vi "总氮总磷质控流程.vi"(0 "队列输入TP":refnum<queue>, 5 "总氮量程切换":enum32{"H", "L", "AUTO"}(ring)=enum."AUTO", 7 "总磷量程切换":enum32{"H", "L", "AUTO"}(ring)=enum."AUTO", 9 "总磷":bool, 11 "总氮":bool) -> (4 "布尔":bool, 6 "总磷中断报警":bool, 8 "总氮中断报警":bool)   [LabVIEW 2016, in "质控单元.lvlib"]
panel:
  out "总磷":bool
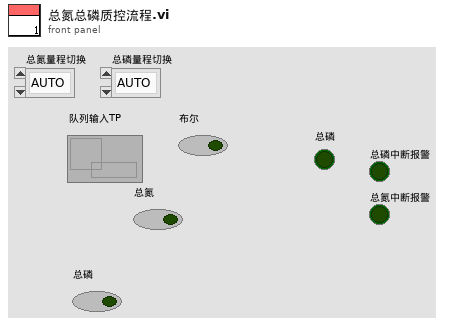
[diagram p1: front panel]
types:
  T1 = enum16{"待机", "启动氨氮水样", "氨氮测量中", "启动氨氮加标", "启动氨氮加标回收", "氨氮加标回收测量中", "启动总氮水样", "总氮测量中", "启动总氮加标", "启动总氮加标回收", "总氮加标回收测量中", "启动总磷水样", "总磷水样测量中", "启动总磷加标", "启动总磷加标回收", "总磷加标回收测量中", "结束"}
  T2 = cluster{"站号":u16, "量程切换":enum32{"H", "L", "AUTO"}, "控制命令":enum16{"启动测量", "标样核查", "零点核查", "跨度核查", "空白测试", "平行样测试", "加标回收", "空白校准", "标样校准", "初始化（清洗）", "停止测试", "仪器重启", "校时", "模式设置", "测量间隔设置"}, "模式设置":enum16{"待机", "连续模式", "周期模式", "定点模式", "受控模式", "手动模式"}, "测量间隔":u16}
  T3 = cluster{"时间标识":timestamp, "设备":string, "日志信息":string}
  T4 = cluster{"系统时间":timestamp, "工作状态":enum16{"空闲", "水样测试", "标样核查", "零点核查", "跨度核查", "空白测试", "平行样测试", "加标回收", "空白校准", "标样校准", "初始化（清洗）"}, "测量模式":enum16{"待机", "连续模式", "周期模式", "定点模式", "受控模式", "手动模式"}, "告警代码":enum16{"无告警", "缺试剂告警", "缺水样告警", "缺蒸馏水告警", "缺标液告警", "仪表漏液告警", "标定异常告警", "超量程告警", "加热异常", "低试剂预警", "超上限告警", "超下限告警", "仪表内部其他异常", "滴定异常告警", "电极异常告警", "量程切换告警", "参数设置告警", "PH电极电位异常", "电导率电极异常", "浊度光度异常", "溶解氧电极异常", "溶解氧光强异常", "温度异常告警", "PH异常告警", "溶解氧异常告警", "电导率异常告警", "浊度异常告警", "叶绿素异常告警", "藻密度异常告警", "蓝绿藻异常告警", "ORP异常告警", "氨氮异常告警", "清洁刷异常告警", "SD卡异常告警", "蓝牙异常告警", "Wifi异常告警", "流程异常告警"}, "故障代码":enum16{"无故障", "电机故障", "温度故障", "通讯故障", "滴定故障"}, "日志代码":u16, "软件版本":u16, "F0":sgl, "F1":sgl, "F2":sgl, "F3":sgl, "T":sgl, "H":sgl, "id":u16, "flowid":u16, "量程":u16, "总磷控温温度1":sgl, "营养盐控温温度2":sgl, "ADC":sgl}
  T5 = enum16{"空闲", "水样测试", "标样核查", "零点核查", "跨度核查", "空白测试", "平行样测试", "加标回收", "空白校准", "标样校准", "初始化（清洗）"}
  T6 = cluster{"因子编码":u32, "单位":u16, "标样参考值":sgl, "水样数据时间":timestamp, "水样实测值":sgl, "水样数据标识":string, "标样数据时间":timestamp, "标样实测值":sgl, "标样数据标识":string, "空白数据时间":timestamp, "空白实测值":sgl, "空白数据标识":string, "零点核查数据时间":timestamp, "零点核查实测值":sgl, "零点核查数据标识":string, "跨度核查数据时间":timestamp, "跨度核查实测值":sgl, "跨度核查数据标识":string, "加标回收数据时间":timestamp, "加标回收实测值":sgl, "加标回收数据标识":string, "平行样数据时间":timestamp, "平行样实测值":sgl, "平行样数据标识":string}
  T7 = cluster{"量程":dbl, "检出限":dbl, "加标前水样浓度":dbl, "加标后水样浓度":dbl, "加标水杯定容体积":dbl, "加标母液浓度":dbl, "加标体积":dbl, "加标回收率":dbl}
  T8 = cluster{"氨氮":u8, "总磷":u8, "总氮":u8, "CODMn":u8, "CODCr":u8}
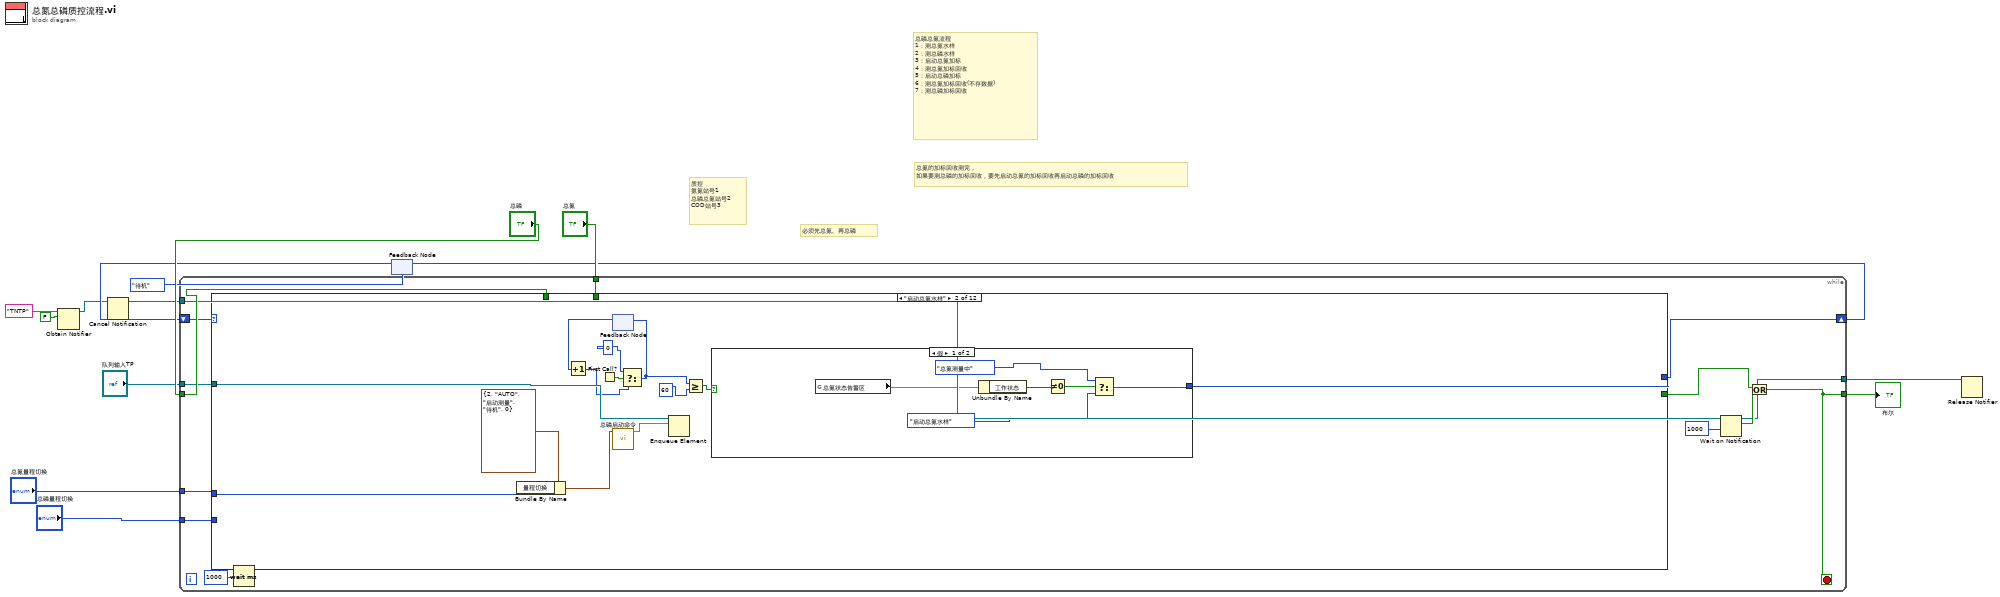
[diagram p0: block diagram]
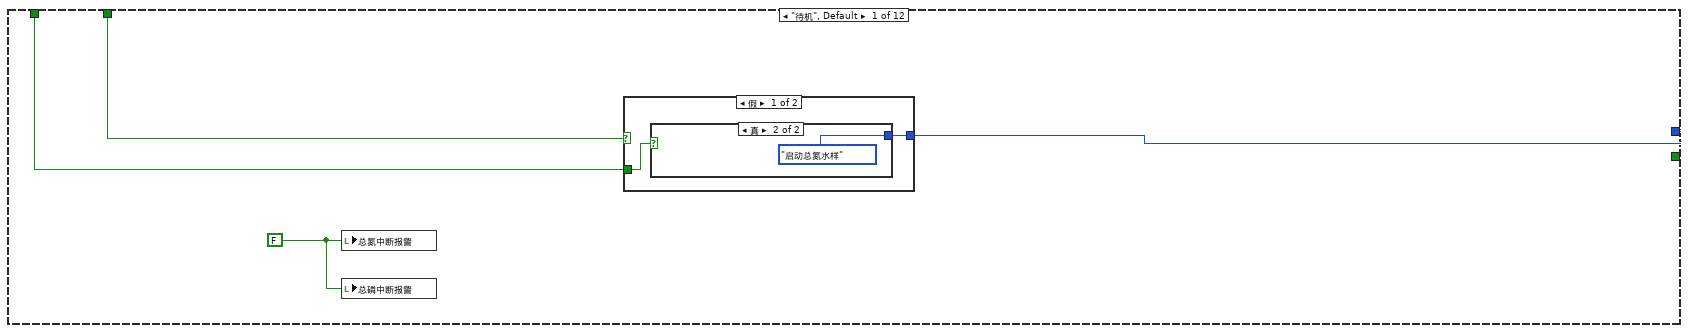
[diagram p2: hidden frame]
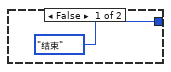
[diagram p3: hidden frame]
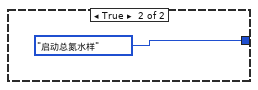
[diagram p4: hidden frame]
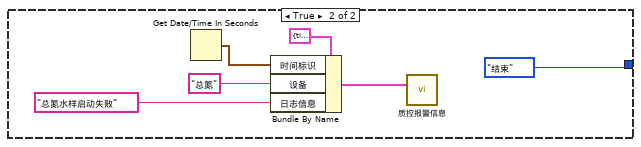
[diagram p5: hidden frame]
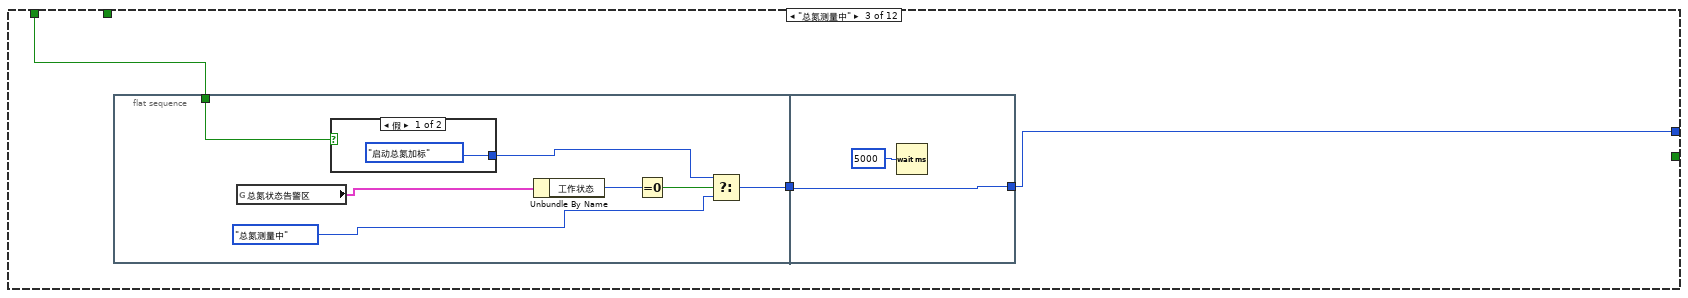
[diagram p6: hidden frame]
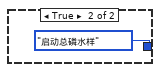
[diagram p7: hidden frame]
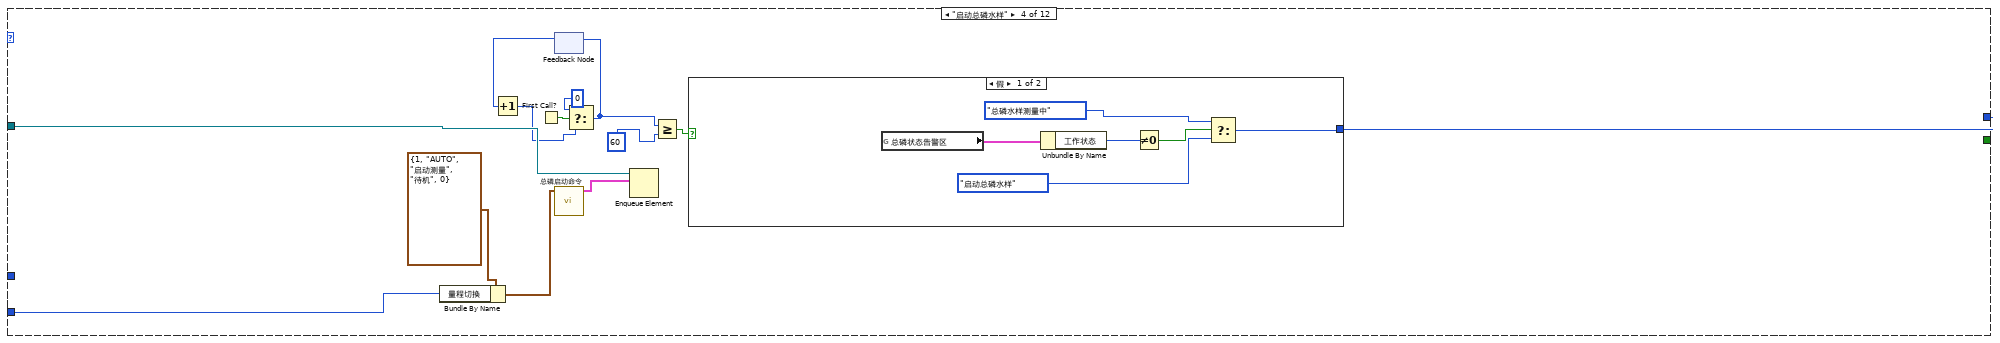
[diagram p8: hidden frame]
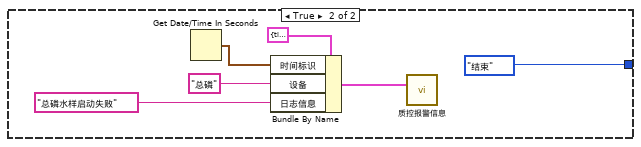
[diagram p9: hidden frame]
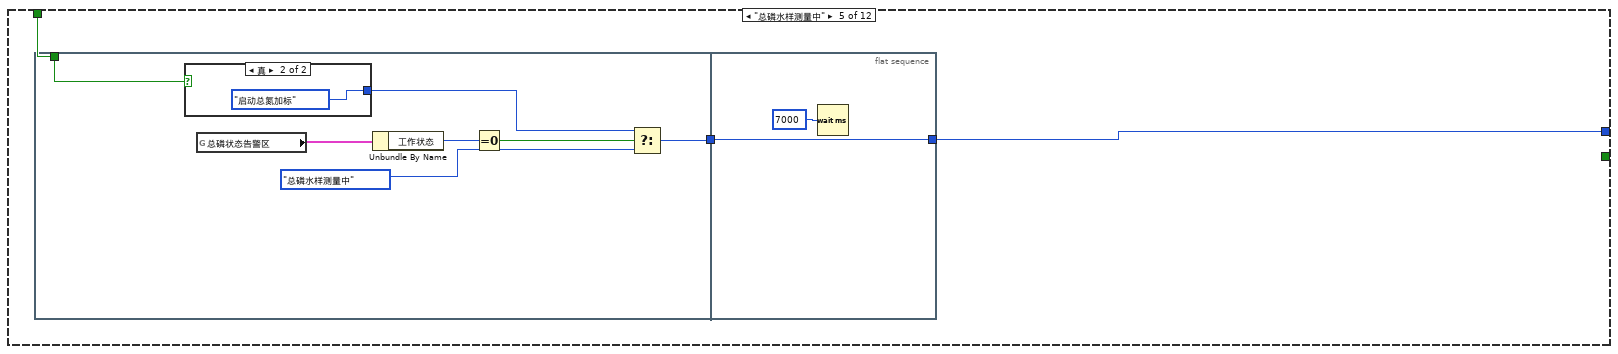
[diagram p10: hidden frame]
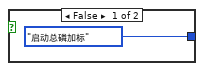
[diagram p11: hidden frame]
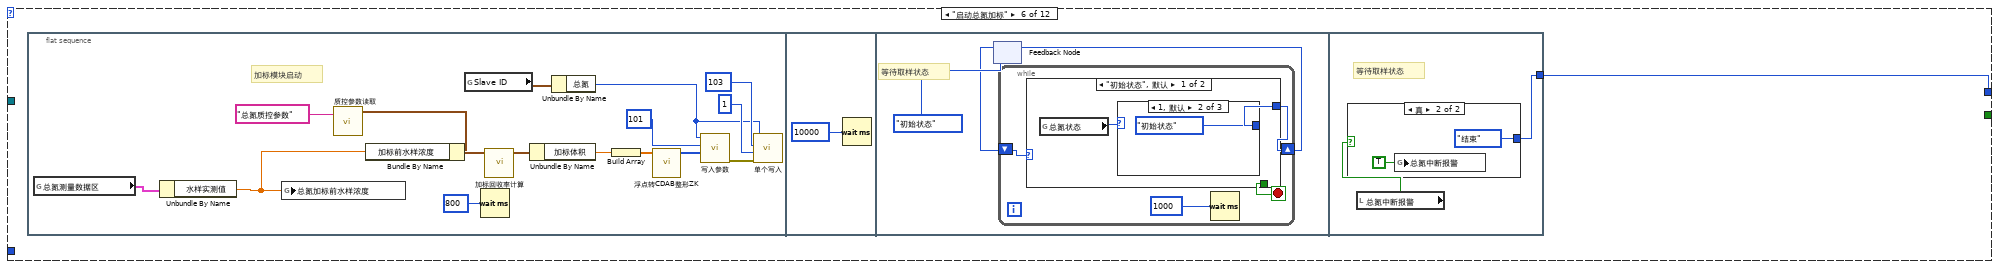
[diagram p12: hidden frame]
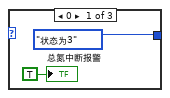
[diagram p13: hidden frame]
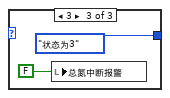
[diagram p14: hidden frame]
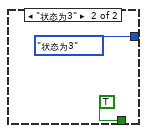
[diagram p15: hidden frame]
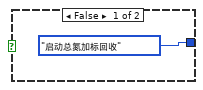
[diagram p16: hidden frame]
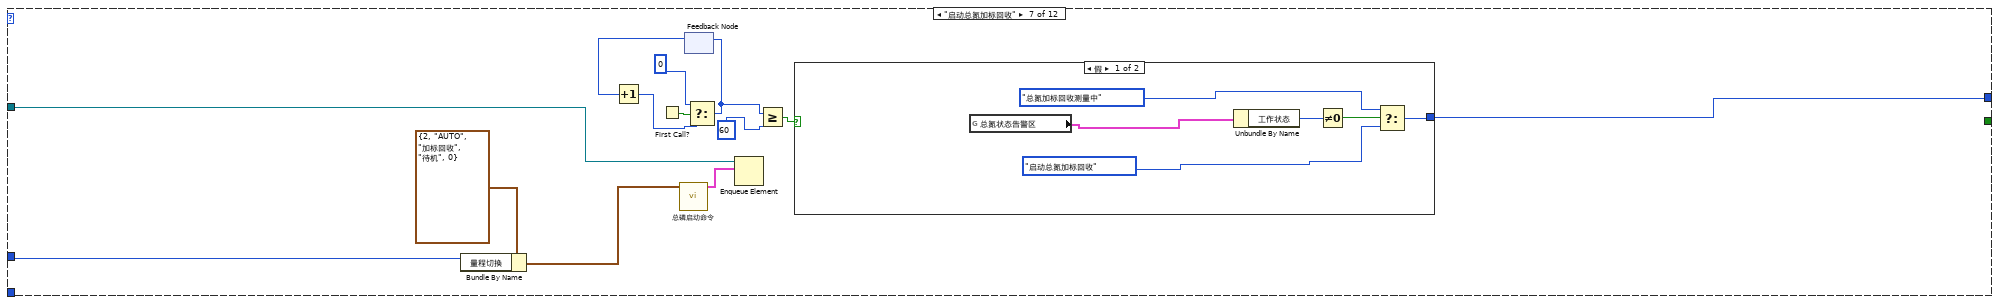
[diagram p17: hidden frame]
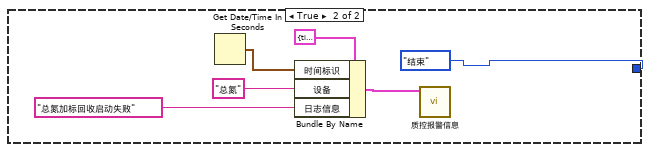
[diagram p18: hidden frame]
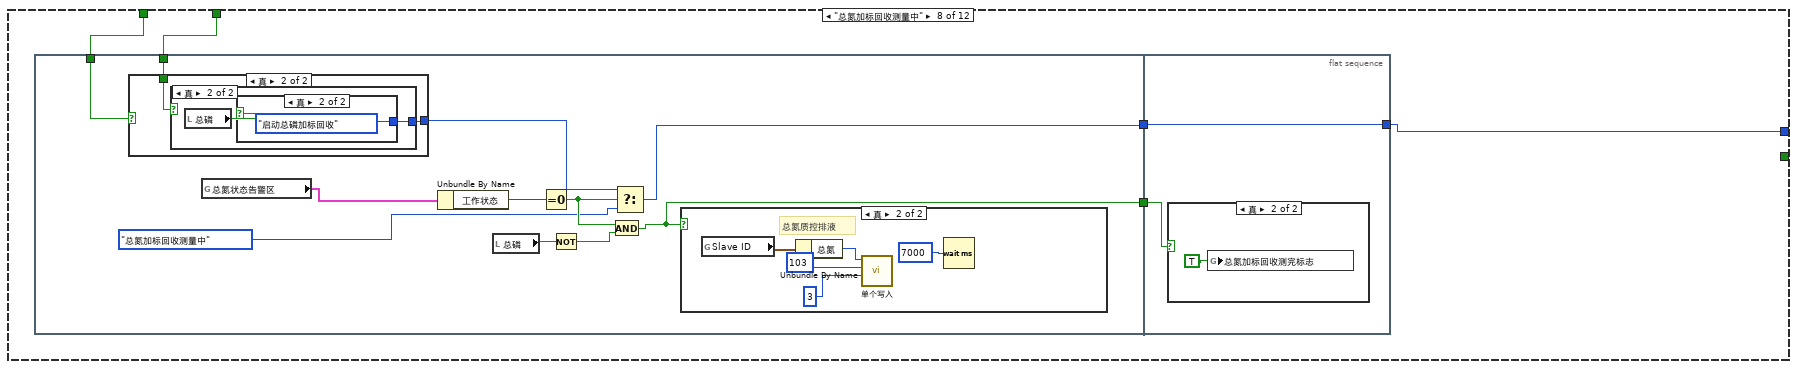
[diagram p19: hidden frame]
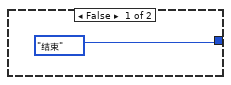
[diagram p20: hidden frame]
diagram:
  # "总磷总氮流程\n1：测总氮水样\n2：测总磷水样\n3：启动总氮加标\n4：测总氮加标回收\n5：启动总磷加标\n6：测总氮加标回收(不存数据)\n7：测总磷加标回收"
  # "总氮的加标回收测完，\n如果要测总磷的加标回收，要先启动总氮的加标回收再启动总磷的加标回收"
  # "质控\n氨氮站号1   \n总磷总氮站号2\nCOD站号3"
  # "必须先总氮、再总磷"
  n1 = Obtain Notifier(name (unnamed)="TNTP" ("名称（未命名）"), notification data type=FALSE) -> (notifier out=w3:refnum<notifier>)  [unwired: 2 in, 2 out]
  n2 = Cancel Notification(0:w3) -> (8:w2:refnum<notifier>)  [unwired: 1 in, 2 out]
  n3 = feedback #1(T1."待机") -> (w6:T1)
  n4 = while {
    tunnel: "队列输入TP" -> [w27]
    tunnel: "总氮" -> [w26]
    tunnel: "总氮量程切换" -> [w24]
    tunnel: "总磷量程切换" -> [w23]
    shift-right: [w25] -> w9
    shift-left: w6 -> [w22]
    tunnel: "总磷" -> [w28]
    tunnel: [w18] -> w13
    tunnel: w2 -> [w17]
    tunnel: [w16] -> w1
    stop <- w18 stop-if-true
    n5 = case shown="\"启动总氮水样\"" w22 {
      tunnel: [w32 w49 w64 w88 w104 w116 w158 w182 w212 w257 w280 T1."结束"] -> w25
      tunnel: w27 -> [_ w50 _ w89 _ _ w160 _ _ w258 _ _]
      tunnel: [_ _ _ _ _ _ _ _ _ _ _ TRUE] -> w19
      tunnel: w28 -> [w31 _ w63 _ _ _ _ w183 _ _ _ _]
      tunnel: w26 -> [w30 _ _ _ w102 _ _ w181 _ _ _ _]
      tunnel: w24 -> [_ w38 _ _ _ _ w155 _ _ _ _ _]
      tunnel: w23 -> [_ _ _ w77 _ _ _ _ _ w253 _ _]
      frame "待机", Default {
        w29 = FALSE ("总氮中断报警")
        n6 = local write "总氮中断报警"(w29) -> ()
        n7 = local write "总磷中断报警"(w29) -> ()
        n8 = case shown="假" w30 {
          tunnel: w31 -> [w33 _]
          tunnel: [w34 T1."启动总氮水样"] -> w32
          frame False {
            n9 = case shown="真" w33 {
              tunnel: [T1."结束" T1."启动总氮水样"] -> w34
              frame False {
              }
              frame True {
              }
            }
          }
          frame True {
          }
        }
      }
      frame "启动总氮水样" {
        n10 = Bundle By Name(cluster=T2 {"站号"=2, "量程切换"=enum."AUTO", "控制命令"=enum."启动测量", "模式设置"=enum."待机", "测量间隔"=0} ("参数"), "量程切换"=w38) -> (w39:T2)
        n11 = First Call?() -> (First Call?: T/F=w47:bool)
        n12 = feedback #2() -> (w46:i32)  [unwired: 1 in]
        n13 = Increment(x=w46) -> (x+1=w45:i32)
        n14 = call "总磷启动命令.vi"("参数"=w39) -> ("启动命令"=w41:cluster{"命令":string, "data":variant})  [unwired: 10 in]
        n15 = Select(t=0, s=w47, f=w45) -> (s? t:f=w44:i32)
        n16 = feedback-in #2(w44) -> ()
        n17 = Enqueue Element(queue=w50, element=w41) -> ()  [unwired: 2 in, 3 out]
        n18 = Greater Or Equal?(x=w44, y=60) -> (x >= y?=w42:bool)
        n19 = case shown="假" w42 {
          tunnel: [w54 T1."结束"] -> w49
          frame False {
            n20 = global read "与总氮交互全局.vi" "总氮状态告警区"() -> (w51:T4)
            n21 = Unbundle By Name(w51) -> ("工作状态"=w55:T5)
            n22 = Not Equal To 0?(x=w55) -> (x != 0?=w56:bool)
            n23 = Select(t=T1."总氮测量中", s=w56, f=T1."启动总氮水样") -> (s? t:f=w54:T1)
          }
          frame True {
            n24 = Get Date/Time In Seconds() -> (seconds since 1Jan1904=w62:timestamp)
            n25 = Bundle By Name(cluster=T3 {"时间标识"=timestamp(0 s since 1904-01-01), "设备"="", "日志信息"=""} ("data in"), "时间标识"=w62, "设备"="总氮", "日志信息"="总氮水样启动失败") -> (w58:T3)
            n26 = call "质控报警信息.vi"("data in"=w58) -> ()  [unwired: 11 in]
          }
        }
      }
      frame "总氮测量中" {
        n27 = flat-sequence {
          tunnel: [w71] -> w65
          tunnel: w63 -> [w67]
          tunnel: [w76] -> w64
          tunnel: w65 -> [w76]
          frame #0 {
            n28 = global read "与总氮交互全局.vi" "总氮状态告警区"() -> (w66:T4)
            n29 = case shown="假" w67 {
              tunnel: [T1."启动总氮加标" T1."启动总磷水样"] -> w69
              frame False {
              }
              frame True {
              }
            }
            n30 = Unbundle By Name(w66) -> ("工作状态"=w72:T5)
            n31 = Equal To 0?(x=w72) -> (x = 0?=w70:bool)
            n32 = Select(t=w69, s=w70, f=T1."总氮测量中") -> (s? t:f=w71:T1)
          }
          frame #1 {
            n33 = Wait (ms)(milliseconds to wait=u32 5000 ("等待时间（毫秒）")) -> ()  [unwired: 1 out]
          }
        }
      }
      frame "启动总磷水样" {
        n34 = Bundle By Name(cluster=T2 {"站号"=1, "量程切换"=enum."AUTO", "控制命令"=enum."启动测量", "模式设置"=enum."待机", "测量间隔"=0} ("参数"), "量程切换"=w77) -> (w78:T2)
        n35 = First Call?() -> (First Call?: T/F=w86:bool)
        n36 = feedback #3() -> (w85:i32)  [unwired: 1 in]
        n37 = Increment(x=w85) -> (x+1=w84:i32)
        n38 = call "总磷启动命令.vi"("参数"=w78) -> ("启动命令"=w80:cluster{"命令":string, "data":variant})  [unwired: 10 in]
        n39 = Select(t=0, s=w86, f=w84) -> (s? t:f=w83:i32)
        n40 = feedback-in #3(w83) -> ()
        n41 = Enqueue Element(queue=w89, element=w80) -> ()  [unwired: 2 in, 3 out]
        n42 = Greater Or Equal?(x=w83, y=60) -> (x >= y?=w81:bool)
        n43 = case shown="假" w81 {
          tunnel: [w92 T1."结束"] -> w88
          frame False {
            n44 = global read "与总磷交互全局.vi" "总磷状态告警区"() -> (w93:T4)
            n45 = Unbundle By Name(w93) -> ("工作状态"=w94:T5)
            n46 = Not Equal To 0?(x=w94) -> (x != 0?=w95:bool)
            n47 = Select(t=T1."总磷水样测量中", s=w95, f=T1."启动总磷水样") -> (s? t:f=w92:T1)
          }
          frame True {
            n48 = Get Date/Time In Seconds() -> (seconds since 1Jan1904=w101:timestamp)
            n49 = Bundle By Name(cluster=T3 {"时间标识"=timestamp(0 s since 1904-01-01), "设备"="", "日志信息"=""} ("data in"), "时间标识"=w101, "设备"="总磷", "日志信息"="总磷水样启动失败") -> (w97:T3)
            n50 = call "质控报警信息.vi"("data in"=w97) -> ()  [unwired: 11 in]
          }
        }
      }
      frame "总磷水样测量中" {
        n51 = flat-sequence {
          tunnel: [w109] -> w103
          tunnel: w102 -> [w106]
          tunnel: [w115] -> w104
          tunnel: w103 -> [w115]
          frame #0 {
            n52 = case shown="真" w106 {
              tunnel: [T1."启动总磷加标" T1."启动总氮加标"] -> w107
              frame False {
              }
              frame True {
              }
            }
            n53 = global read "与总磷交互全局.vi" "总磷状态告警区"() -> (w110:T4)
            n54 = Unbundle By Name(w110) -> ("工作状态"=w111:T5)
            n55 = Equal To 0?(x=w111) -> (x = 0?=w108:bool)
            n56 = Select(t=w107, s=w108, f=T1."总磷水样测量中") -> (s? t:f=w109:T1)
          }
          frame #1 {
            n57 = Wait (ms)(milliseconds to wait=u32 7000 ("等待时间（毫秒）")) -> ()  [unwired: 1 out]
          }
        }
      }
      frame "启动总氮加标" {
        n58 = flat-sequence {
          tunnel: [w151] -> w116
          frame #0 {
            # "加标模块启动"
            n59 = global read "与总氮交互全局.vi" "总氮测量数据区"() -> (w119:T6)
            n60 = Unbundle By Name(w119) -> ("水样实测值"=w120:sgl)
            n61 = global write "水样浓度全局.vi" "总氮加标前水样浓度"(w120) -> ()
            n62 = call "质控参数读取.vi"("section"="总氮质控参数") -> ("参数"=w122:T7)  [unwired: 9 in, 1 out]
            n63 = Bundle By Name(cluster=w122, "加标前水样浓度"=w120) -> (w131:T7)
            n64 = global read "断电保存全局.vi" "Slave ID"() -> (w118:T8)
            n65 = Wait (ms)(milliseconds to wait=u32 800 ("等待时间（毫秒）")) -> ()  [unwired: 1 out]
            n66 = call "加标回收率计算.vi"("参数"=w131) -> ("参数 out"=w130:T7)  [unwired: 9 in, 1 out]
            n67 = Unbundle By Name(w130) -> ("加标体积"=w123:dbl)
            n68 = Unbundle By Name(w118) -> ("总氮"=w117:u8)
            n69 = Build Array(w123) -> (w129:dbl[])
            n70 = call "浮点转CDAB整形ZK.vi"("浮点数"=w129) -> ("CDAB整形输出"=w124:u16[])  [unwired: 10 in]
            n71 = call "写入参数.vi"("values"=w124, "starting address"=u16 101, "Slave ID"=w117) -> ("error out"=w128:errorcluster)  [unwired: 8 in]
            n72 = call "单个写入.vi"("Error in"=w128, "value"=u16 1, "address"=u16 103, "Slave ID"=w117) -> ()  [unwired: 7 in, 1 out]
          }
          frame #1 {
            n73 = Wait (ms)(milliseconds to wait=u32 10000 ("等待时间（毫秒）")) -> ()  [unwired: 1 out]
          }
          frame #2 {
            # "等待取样状态"
            n74 = feedback #4(enum16{"初始状态", "状态为3"}."初始状态") -> (w135:enum16{"初始状态", "状态为3"})
            n75 = while {
              shift-right: [w139] -> w134
              shift-left: w135 -> [w140]
              stop <- w138 stop-if-true
              n76 = case shown="\"初始状态\", 默认" w140 {
                tunnel: [w142 enum16{"初始状态", "状态为3"}."状态为3"] -> w139
                tunnel: [_ TRUE] -> w138
                frame "初始状态", Default {
                  n77 = global read "加标回收状态全局变量.vi" "总氮状态"() -> (w141:u16)
                  n78 = case shown="1, 默认" w141 {
                    tunnel: [enum16{"初始状态", "状态为3"}."状态为3" enum16{"初始状态", "状态为3"}."初始状态" enum16{"初始状态", "状态为3"}."状态为3"] -> w142
                    frame 0 {
                      "总氮中断报警" <- TRUE ("总氮中断报警")
                    }
                    frame 1, Default {
                    }
                    frame 3 {
                      n79 = local write "总氮中断报警"(FALSE ("总氮中断报警")) -> ()
                    }
                  }
                }
                frame "状态为3" {
                }
              }
              n80 = Wait (ms)(milliseconds to wait=u32 1000 ("等待时间（毫秒）")) -> ()  [unwired: 1 out]
            }
            n81 = feedback-in #4(w134) -> ()
          }
          frame #3 {
            # "等待取样状态"
            n82 = local read "总氮中断报警"() -> (w150:bool)
            n83 = case shown="真" w150 {
              tunnel: [T1."启动总氮加标回收" T1."结束"] -> w151
              frame False {
              }
              frame True {
                n84 = global write "质控中断报警全局.vi" "总氮中断报警"(TRUE ("总氮中断报警")) -> ()
              }
            }
          }
        }
      }
      frame "启动总氮加标回收" {
        n85 = Bundle By Name(cluster=T2 {"站号"=2, "量程切换"=enum."AUTO", "控制命令"=enum."加标回收", "模式设置"=enum."待机", "测量间隔"=0} ("参数"), "量程切换"=w155) -> (w156:T2)
        n86 = First Call?() -> (First Call?: T/F=w166:bool)
        n87 = call "总磷启动命令.vi"("参数"=w156) -> ("启动命令"=w159:cluster{"命令":string, "data":variant})  [unwired: 10 in]
        n88 = feedback #5() -> (w165:i32)  [unwired: 1 in]
        n89 = Increment(x=w165) -> (x+1=w164:i32)
        n90 = Select(t=0, s=w166, f=w164) -> (s? t:f=w163:i32)
        n91 = feedback-in #5(w163) -> ()
        n92 = Enqueue Element(queue=w160, element=w159) -> ()  [unwired: 2 in, 3 out]
        n93 = Greater Or Equal?(x=w163, y=60) -> (x >= y?=w161:bool)
        n94 = case shown="假" w161 {
          tunnel: [w171 T1."结束"] -> w158
          frame False {
            n95 = global read "与总氮交互全局.vi" "总氮状态告警区"() -> (w168:T4)
            n96 = Unbundle By Name(w168) -> ("工作状态"=w173:T5)
            n97 = Not Equal To 0?(x=w173) -> (x != 0?=w172:bool)
            n98 = Select(t=T1."总氮加标回收测量中", s=w172, f=T1."启动总氮加标回收") -> (s? t:f=w171:T1)
          }
          frame True {
            n99 = Get Date/Time In Seconds() -> (seconds since 1Jan1904=w179:timestamp)
            n100 = Bundle By Name(cluster=T3 {"时间标识"=timestamp(0 s since 1904-01-01), "设备"="", "日志信息"=""} ("data in"), "时间标识"=w179, "设备"="总氮", "日志信息"="总氮加标回收启动失败") -> (w175:T3)
            n101 = call "质控报警信息.vi"("data in"=w175) -> ()  [unwired: 11 in]
          }
        }
      }
      frame "总氮加标回收测量中" {
        n102 = flat-sequence {
          tunnel: [w194] -> w184
          tunnel: w183 -> [w191]
          tunnel: w181 -> [w187]
          tunnel: [w185] -> w180
          tunnel: [w210] -> w182
          tunnel: w184 -> [w210]
          tunnel: w180 -> [w209]
          frame #0 {
            n103 = case shown="真" w191 {
              tunnel: [T1."结束" w198] -> w193
              tunnel: w187 -> [_ w197]
              frame False {
              }
              frame True {
                n104 = case shown="真" w197 {
                  tunnel: [T1."启动总磷加标回收" w201] -> w198
                  frame False {
                  }
                  frame True {
                    n105 = local read "总磷"() -> (w200:bool)
                    n106 = case shown="真" w200 {
                      tunnel: [T1."启动总磷加标" T1."启动总磷加标回收"] -> w201
                      frame False {
                      }
                      frame True {
                      }
                    }
                  }
                }
              }
            }
            n107 = global read "与总氮交互全局.vi" "总氮状态告警区"() -> (w186:T4)
            n108 = Unbundle By Name(w186) -> ("工作状态"=w195:T5)
            n109 = local read "总磷"() -> (w189:bool)
            n110 = Equal To 0?(x=w195) -> (x = 0?=w192:bool)
            n111 = Not(x=w189) -> (.not. x?=w188:bool)
            n112 = And(x=w192, y=w188) -> (x .and. y?=w185:bool)
            n113 = Select(t=w193, s=w192, f=T1."总氮加标回收测量中") -> (s? t:f=w194:T1)
            n114 = case shown="真" w185 {
              frame False {
              }
              frame True {
                # "总氮质控排液"
                n115 = global read "断电保存全局.vi" "Slave ID"() -> (w205:T8)
                n116 = Unbundle By Name(w205) -> ("总氮"=w204:u8)
                n117 = call "单个写入.vi"("value"=u16 3, "address"=u16 103, "Slave ID"=w204) -> ()  [unwired: 8 in, 1 out]
                n118 = Wait (ms)(milliseconds to wait=u32 7000 ("等待时间（毫秒）")) -> ()  [unwired: 1 out]
              }
            }
          }
          frame #1 {
            n119 = case shown="真" w209 {
              frame False {
              }
              frame True {
                n120 = global write "质控测完标志全局 1.vi" "总氮加标回收测完标志"(TRUE) -> ()
              }
            }
          }
        }
      }
      frame "启动总磷加标" {
        n121 = flat-sequence {
          tunnel: [w249] -> w212
          frame #0 {
            n122 = Wait (ms)(milliseconds to wait=u32 180000 ("等待时间（毫秒）")) -> ()  [unwired: 1 out]
          }
          frame #1 {
            # "加标模块启动"
            n123 = global read "与总磷交互全局.vi" "总磷测量数据区"() -> (w217:T6)
            n124 = Unbundle By Name(w217) -> ("水样实测值"=w216:sgl)
            n125 = call "质控参数读取.vi"("section"="总磷质控参数") -> ("参数"=w219:T7)  [unwired: 9 in, 1 out]
            n126 = Bundle By Name(cluster=w219, "加标前水样浓度"=w216) -> (w228:T7)
            n127 = global write "水样浓度全局.vi" "总磷加标前水样浓度"(w216) -> ()
            n128 = Wait (ms)(milliseconds to wait=u32 800 ("等待时间（毫秒）")) -> ()  [unwired: 1 out]
            n129 = call "加标回收率计算.vi"("参数"=w228) -> ("参数 out"=w227:T7)  [unwired: 9 in, 1 out]
            n130 = global read "断电保存全局.vi" "Slave ID"() -> (w215:T8)
            n131 = Unbundle By Name(w227) -> ("加标体积"=w220:dbl)
            n132 = Unbundle By Name(w215) -> ("总磷"=w214:u8)
            n133 = Build Array(w220) -> (w226:dbl[])
            n134 = call "浮点转CDAB整形ZK.vi"("浮点数"=w226) -> ("CDAB整形输出"=w221:u16[])  [unwired: 10 in]
            n135 = call "写入参数.vi"("values"=w221, "starting address"=u16 101, "Slave ID"=w214) -> ("error out"=w225:errorcluster)  [unwired: 8 in]
            n136 = call "单个写入.vi"("Error in"=w225, "value"=u16 1, "address"=u16 103, "Slave ID"=w214) -> ()  [unwired: 7 in, 1 out]
          }
          frame #2 {
            n137 = Wait (ms)(milliseconds to wait=u32 10000 ("等待时间（毫秒）")) -> ()  [unwired: 1 out]
          }
          frame #3 {
            # "等待取样状态"
            n138 = feedback #6(enum16{"初始状态", "状态为3"}."初始状态") -> (w232:enum16{"初始状态", "状态为3"})
            n139 = while {
              shift-right: [w236] -> w231
              shift-left: w232 -> [w237]
              stop <- w235 stop-if-true
              n140 = case shown="\"状态为3\"" w237 {
                tunnel: [w239 enum16{"初始状态", "状态为3"}."状态为3"] -> w236
                tunnel: [_ TRUE] -> w235
                frame "初始状态", Default {
                  n141 = global read "加标回收状态全局变量.vi" "总磷状态"() -> (w238:u16)
                  n142 = case shown="0" w238 {
                    tunnel: [enum16{"初始状态", "状态为3"}."状态为3" enum16{"初始状态", "状态为3"}."初始状态" enum16{"初始状态", "状态为3"}."状态为3"] -> w239
                    frame 0 {
                      "总磷中断报警" <- TRUE ("总磷中断报警")
                    }
                    frame 1, Default {
                    }
                    frame 3 {
                      n143 = local write "总磷中断报警"(FALSE ("总磷中断报警")) -> ()
                    }
                  }
                }
                frame "状态为3" {
                  "总磷" <- TRUE
                }
              }
              n144 = Wait (ms)(milliseconds to wait=u32 1000 ("等待时间（毫秒）")) -> ()  [unwired: 1 out]
            }
            n145 = feedback-in #6(w231) -> ()
          }
          frame #4 {
            n146 = local read "总磷中断报警"() -> (w248:bool)
            n147 = case shown="真" w248 {
              tunnel: [T1."启动总氮加标回收" T1."结束"] -> w249
              frame False {
                # "等待取样状态"
              }
              frame True {
                n148 = global write "质控中断报警全局.vi" "总磷中断报警"(TRUE ("总磷中断报警")) -> ()
              }
            }
          }
        }
      }
      frame "启动总磷加标回收" {
        n149 = Bundle By Name(cluster=T2 {"站号"=1, "量程切换"=enum."AUTO", "控制命令"=enum."加标回收", "模式设置"=enum."待机", "测量间隔"=0} ("参数"), "量程切换"=w253) -> (w254:T2)
        n150 = First Call?() -> (First Call?: T/F=w265:bool)
        n151 = feedback #7() -> (w264:i32)  [unwired: 1 in]
        n152 = Increment(x=w264) -> (x+1=w263:i32)
        n153 = call "总磷启动命令.vi"("参数"=w254) -> ("启动命令"=w259:cluster{"命令":string, "data":variant})  [unwired: 10 in]
        n154 = Select(t=0, s=w265, f=w263) -> (s? t:f=w262:i32)
        n155 = feedback-in #7(w262) -> ()
        n156 = Enqueue Element(queue=w258, element=w259) -> ()  [unwired: 2 in, 3 out]
        n157 = Greater Or Equal?(x=w262, y=60) -> (x >= y?=w260:bool)
        n158 = case shown="真" w260 {
          tunnel: [w269 T1."结束"] -> w257
          frame False {
            n159 = global read "与总磷交互全局.vi" "总磷状态告警区"() -> (w270:T4)
            n160 = Unbundle By Name(w270) -> ("工作状态"=w271:T5)
            n161 = Not Equal To 0?(x=w271) -> (x != 0?=w272:bool)
            n162 = Select(t=T1."总磷加标回收测量中", s=w272, f=T1."启动总磷加标回收") -> (s? t:f=w269:T1)
          }
          frame True {
            n163 = Get Date/Time In Seconds() -> (seconds since 1Jan1904=w278:timestamp)
            n164 = Bundle By Name(cluster=T3 {"时间标识"=timestamp(0 s since 1904-01-01), "设备"="", "日志信息"=""} ("data in"), "时间标识"=w278, "设备"="总磷", "日志信息"="总磷加标回收启动失败") -> (w274:T3)
            n165 = call "质控报警信息.vi"("data in"=w274) -> ()  [unwired: 11 in]
          }
        }
        n166 = local write "总磷"(FALSE ("总磷")) -> ()
      }
      frame "总磷加标回收测量中" {
        n167 = flat-sequence {
          tunnel: [w285] -> w281
          tunnel: [w282] -> w279
          tunnel: [w294] -> w280
          tunnel: w281 -> [w294]
          tunnel: w279 -> [w293]
          frame #0 {
            n168 = global read "与总磷交互全局.vi" "总磷状态告警区"() -> (w286:T4)
            n169 = Unbundle By Name(w286) -> ("工作状态"=w287:T5)
            n170 = Equal To 0?(x=w287) -> (x = 0?=w282:bool)
            n171 = Select(t=T1."结束", s=w282, f=T1."总磷加标回收测量中") -> (s? t:f=w285:T1)
            n172 = case shown="真" w282 {
              frame False {
              }
              frame True {
                # "总磷质控排液"
                n173 = global read "断电保存全局.vi" "Slave ID"() -> (w289:T8)
                n174 = Wait (ms)(milliseconds to wait=u32 5000 ("等待时间（毫秒）")) -> ()  [unwired: 1 out]
                n175 = Unbundle By Name(w289) -> ("总磷"=w288:u8)
                n176 = call "单个写入.vi"("value"=u16 3, "address"=u16 103, "Slave ID"=w288) -> ()  [unwired: 8 in, 1 out]
              }
            }
          }
          frame #1 {
            n177 = case shown="真" w293 {
              frame False {
              }
              frame True {
                n178 = global write "质控测完标志全局 1.vi" "总磷加标回收测完标志"(TRUE) -> ()
              }
            }
          }
        }
      }
      frame "结束" {
        n179 = Wait (ms)(milliseconds to wait=u32 5000 ("等待时间（毫秒）")) -> ()  [unwired: 1 out]
      }
    }
    n180 = Wait (ms)(milliseconds to wait=u32 1000 ("等待时间（毫秒）")) -> ()  [unwired: 1 out]
    n181 = Wait on Notification(notifier=w17, timeout in ms (-1)=1000 ("超时毫秒(-1)")) -> (notifier out=w16:refnum<notifier>, notification=w20:bool)  [unwired: 2 in, 2 out]
    n182 = Or(x=w19, y=w20) -> (x .or. y?=w18:bool)
  }
  "布尔" <- w13
  n183 = feedback-in #1(w9) -> ()
  n184 = Release Notifier(notifier=w1) -> ()  [unwired: 2 in, 3 out]
